vi "Spectrum_Main.vi"() -> ()   [LabVIEW 2021]
uses:
  Sources/Plotting-Axis.ctl
  GEN_States.ctl
  Sources/Config_Cluster.ctl
  Sources/Mode_Enum.ctl
  Sources/Data_Cluster.ctl
  Sources/Measurement_Cluster.ctl
  VISAS.ctl
  1375486a-d526-4950-a4e9-ede105372d37.vi
  <vilib>/Utility/config.llb/NI_LVConfig.lvlib
panel:
  in  "Control Tab":enum32{"General", "Scope/Gen", "VNA", "Configs"}(tab)
  out "VNA":bool
  out "Generator":bool
  in  "StopM_Button":bool
  in  "Log_Button":bool
  in  "Measure_Button":bool
  out "Globals":bool
  out "Scope":bool
  out "Logging":bool
  out "Measuring":bool
  out "Magnetic Field":dbl
  out "Temperature":dbl
  in  "Offset (V)":dbl
  in  "Amplitude (Vpp)":dbl
  in  "Frequency (Hz)":dbl
  in  "SendSet_scopgen_Button":bool
  in  "Refresh_scopgen_Button":bool
  in  "Vertical Scale (V/div)":dbl
  in  "Horizontal Scale (1/t)":dbl
  in  "Tab Control":enum32{"Scope", "Gen"}(tab)
  in  "Scope Channel":enum16{"Channel 1", "Channel 2"}(ring)
  in  "RTC1002 VISA COM":refnum<visa-resource-name>
  in  "Gen VISA COM":refnum<visa-resource-name>
  in  "LoadConfig_Button":bool
  in  "ApplyConfig_Button":bool
  in  "SaveConfig_Button":bool
  in  "Retry_Button":bool
  in  "Config Path (Blank is default)":path
  in  "Global Temp VAR":refnum<k21>
  in  "Global Mag VAR":refnum<k21>
  in  "Logging Path":path
  in  "Display Tab":T1(tab)
  out "Status":string
  in  "Clear_Button":bool
  in  "Y-Axis":T2
  in  "X-Axis":T2
  out "Test Graph":cluster{"X":dbl, "Y":dbl}[](graph)
  in  "Max Elements":i32=5000
  out "Scope Display":waveform(dbl)(graph)
  in  "Exit_Button":bool
  # "Instrument Settings"
  # "Global Var. Settings"
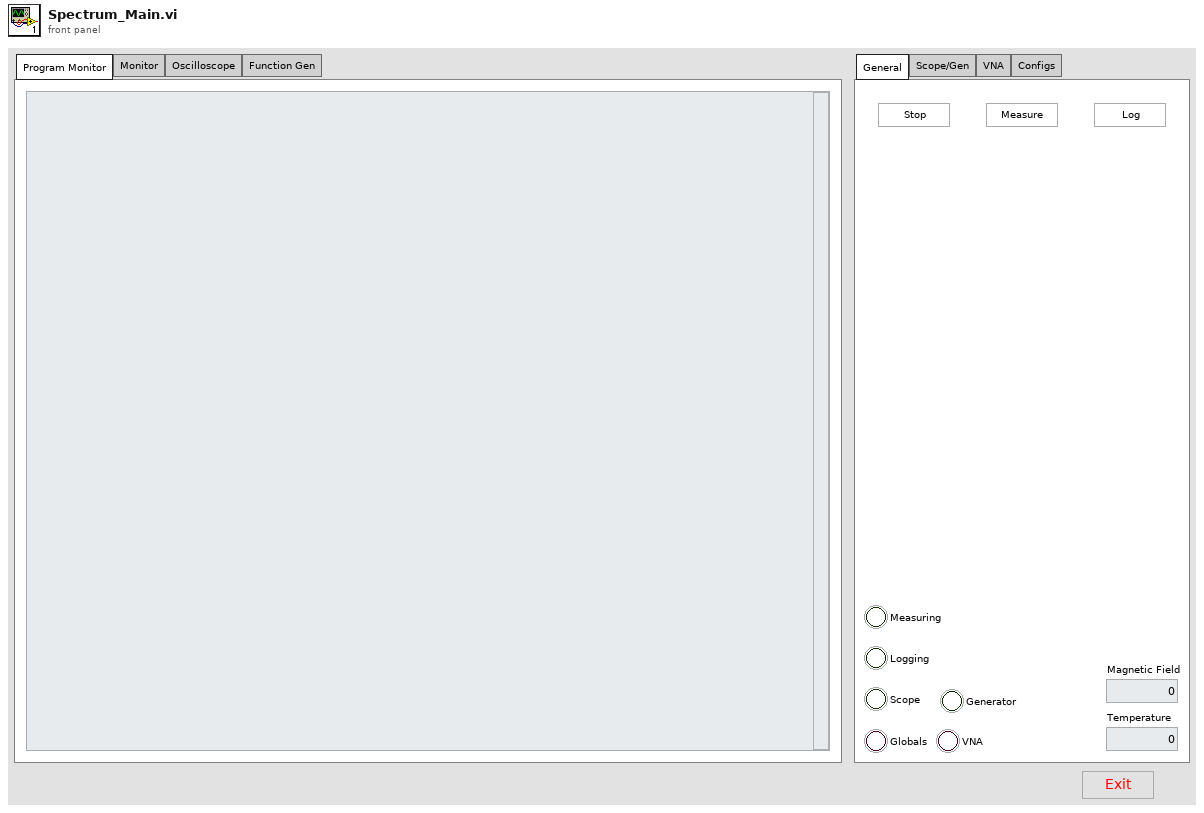
[diagram p1: front panel]
types:
  T1 = enum32{"Program Monitor", "Monitor", "Oscilloscope", "Function Gen"}
  T2 = typedef "Plotting-Axis.ctl" = enum16{"Time", "Temperature", "MagneticField", "Capacitance", "Loss"}
  T3 = typedef "GEN_States.ctl" = enum16{"SetupSettings", "GetSettings", "SetupInstruments", "SetupGEN", "SetupVNA", "ClearBuffers", "SwitchToMeas", "SwitchToLog", "SwitchToOff", "Disconnect", "ApplyConfig", "ExitSafe", "RefreshPlotMUnits", "UpdatePlots", "RefreshMUnits", "Read/WriteAll", "RetryComs", "SendSettings", "InitGUI", "RefreshGUI", "ComsFail", "SaveConfig", "Idle", "ProgInit"}
  T4 = typedef "VISAS.ctl" = cluster{"Gen VISA":refnum<visa-resource-name>, "RTC1002 VISA":refnum<visa-resource-name>, "VNA VISA":refnum<visa-resource-name>}
  T5 = typedef "Data_Cluster.ctl" = cluster{"Value":dbl, "GUI Data Cluster":cluster{"SBR":u16}, "Timing":cluster{"Last Operation":dbl}, "Measurements":T6[], "Scope Capture":waveform(dbl)}
  T6 = typedef "Measurement_Cluster.ctl" = cluster{"Time Stamp":timestamp, "Cap":dbl, "Temperature":dbl, "MagneticField":dbl, "Loss":dbl, "ExVoltage":dbl, "Error":dbl}
  T7 = typedef "Config_Cluster.ctl" = cluster{"General":cluster{"Config.ini":path, "Default Logging Path":path}, "Hardware":cluster{"Global T VAR":refnum<k21>, "Global B VAR":refnum<k21>, "VISAS":cluster{"GEN COM":refnum<visa-resource-name>, "SCOPE COM":refnum<visa-resource-name>, "VNA COM":refnum<visa-resource-name>}, "Connected?":cluster{"SCOPE":bool, "GEN":bool, "VNA":bool}}, "Operation":cluster{"Operation Mode":T8, "Status":string, "NewLog?":bool, "OvenWarn":bool, "Scope Settings":cluster{"TimeBase":dbl, "VerticalScale":dbl, "Channel":enum16{"Channel 2", "Channel 1"}}, "Gen Settings":cluster{"Amplitude":dbl, "Frequency":dbl, "Offset":dbl}}}
  T8 = typedef "Mode_Enum.ctl" = enum16{"Logging", "Idle-Off", "Idle"}
  T9 = cluster{"Scope":refnum<vi>, "Generator":refnum<vi>, "VNA":refnum<vi>}
  T10 = typedef "NI_LVConfig.lvlib/Config Data RefNum.ctl" = refnum<k1>
  T11 = cluster{"GEN COM":refnum<visa-resource-name>, "SCOPE COM":refnum<visa-resource-name>, "VNA COM":refnum<visa-resource-name>}
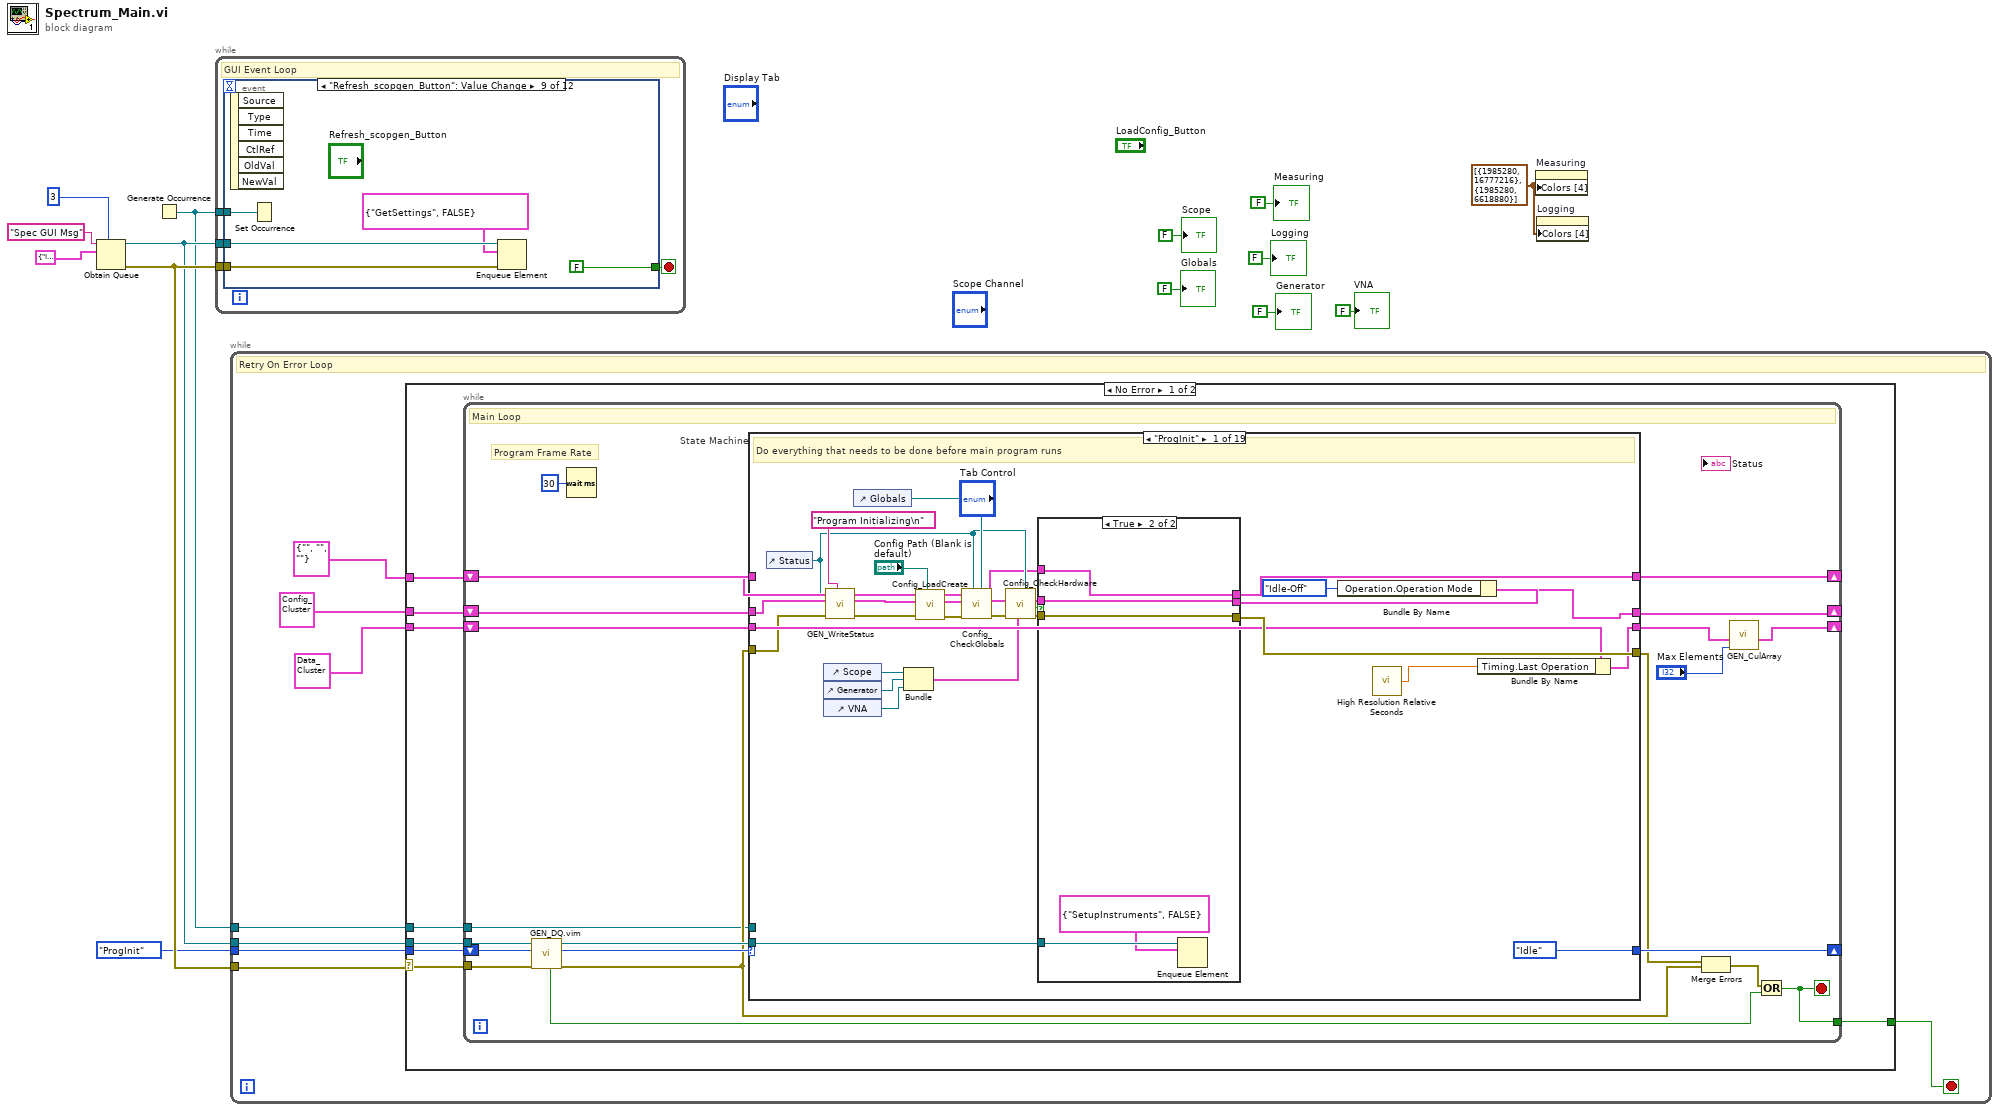
[diagram p0: block diagram]
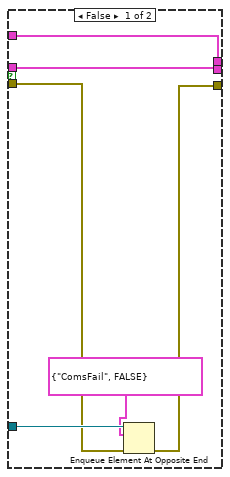
[diagram p2: hidden frame]
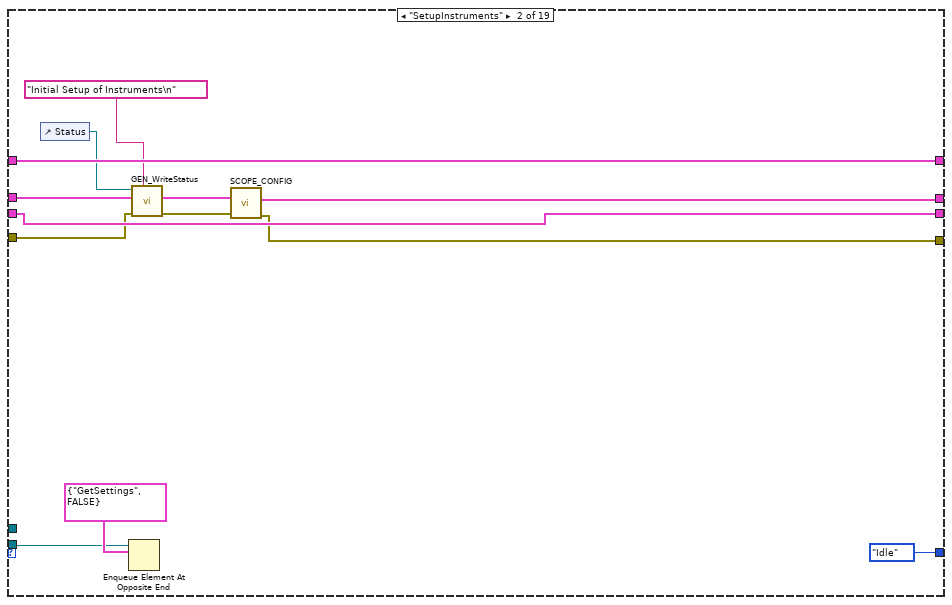
[diagram p3: hidden frame]
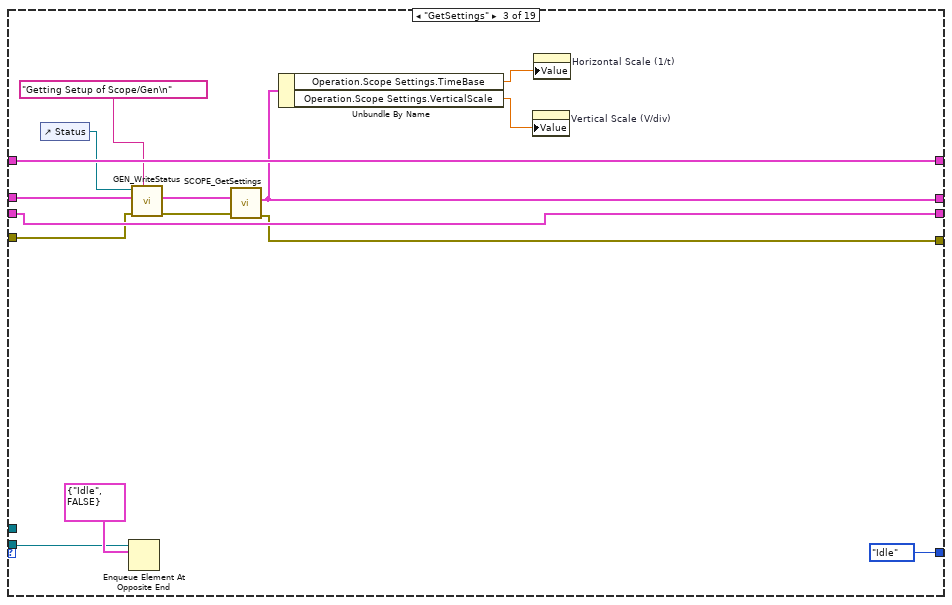
[diagram p4: hidden frame]
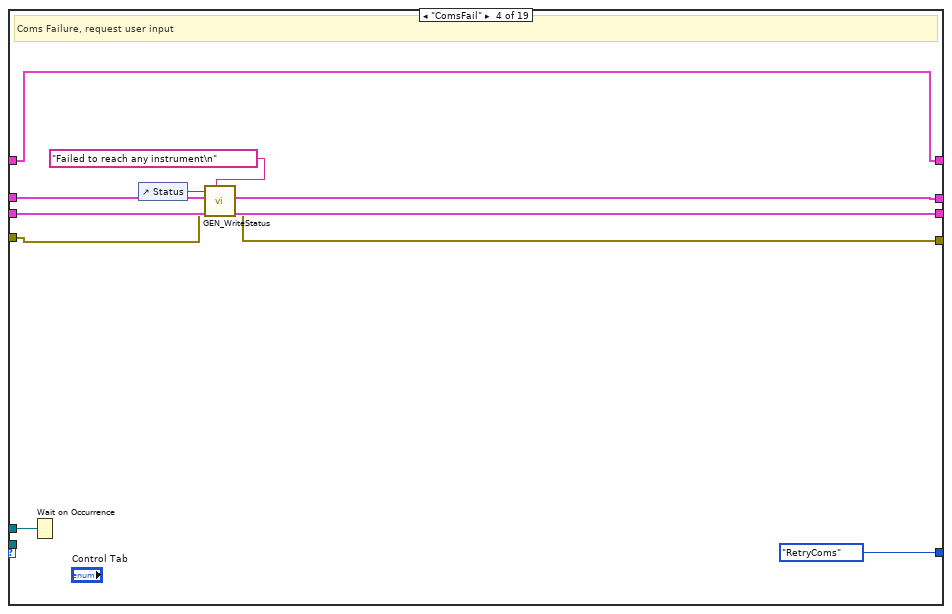
[diagram p5: hidden frame]
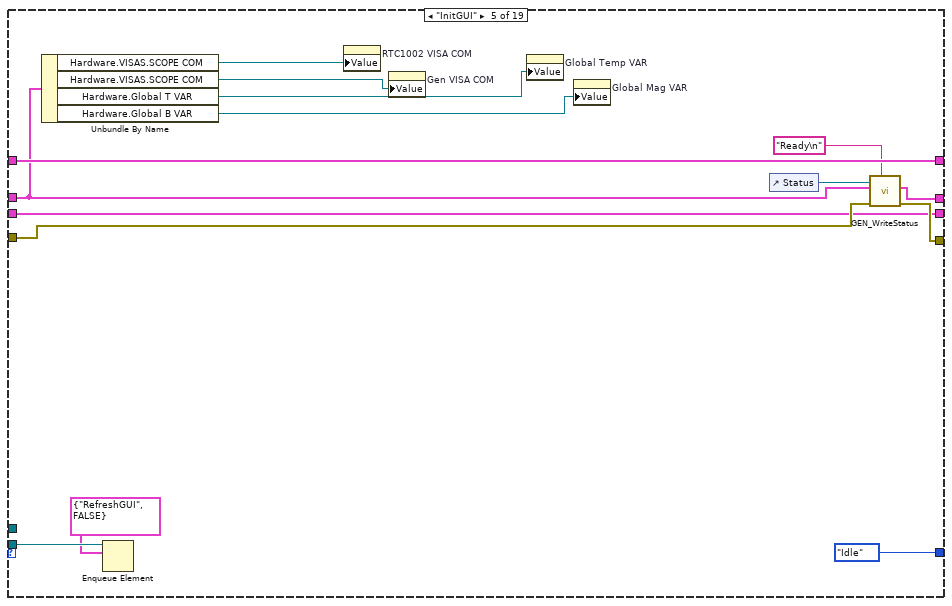
[diagram p6: hidden frame]
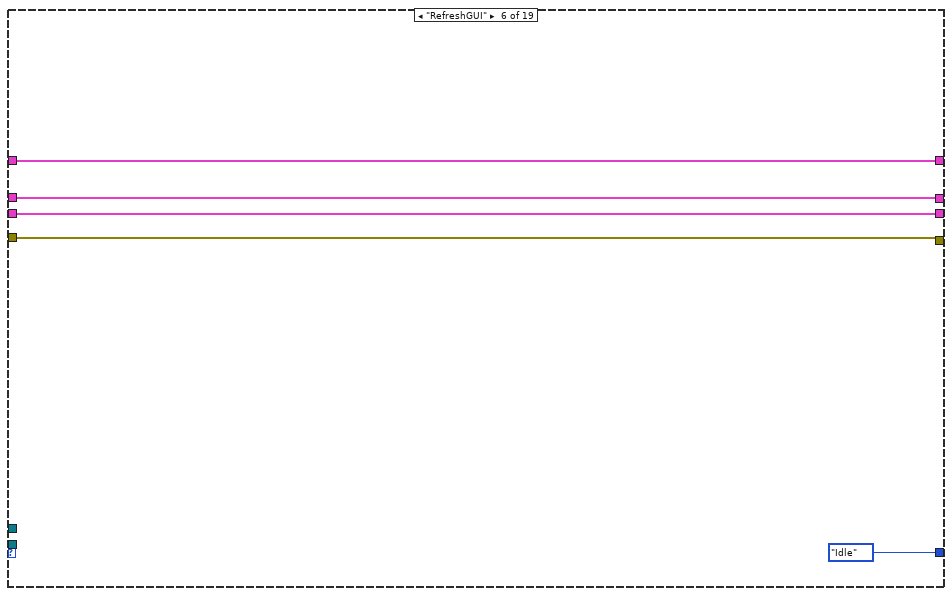
[diagram p7: hidden frame]
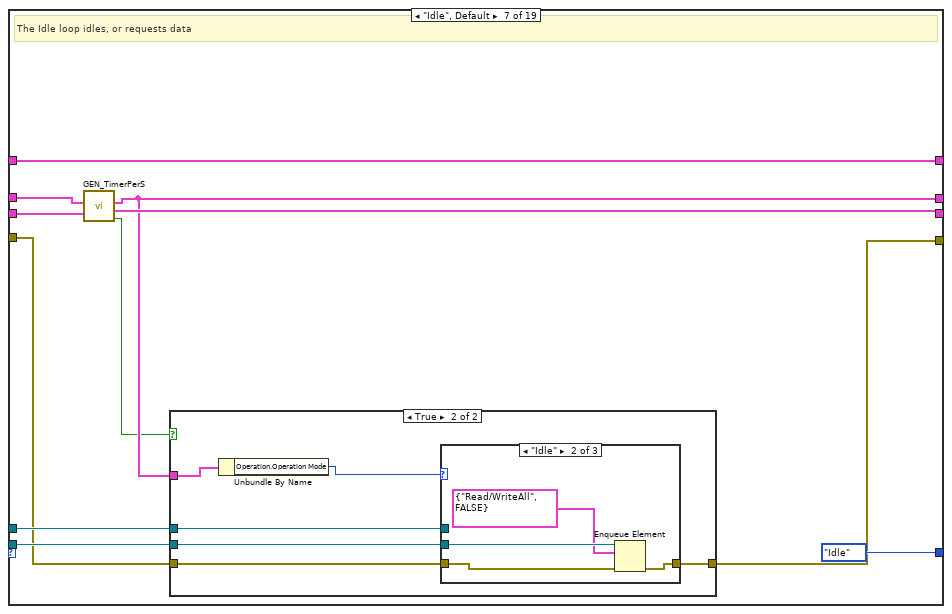
[diagram p8: hidden frame]
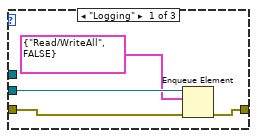
[diagram p10: hidden frame]
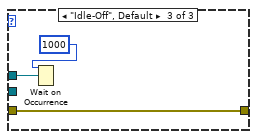
[diagram p11: hidden frame]
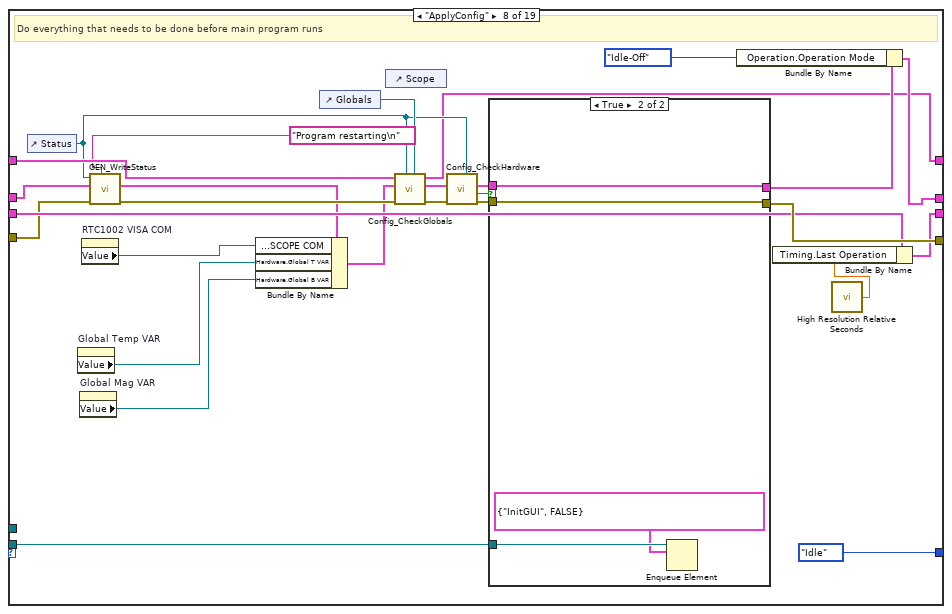
[diagram p12: hidden frame]
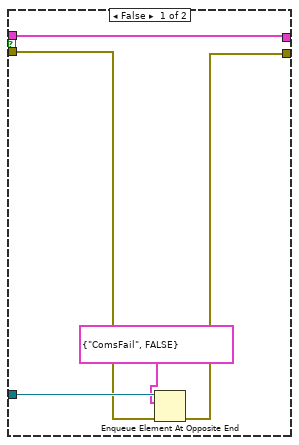
[diagram p13: hidden frame]
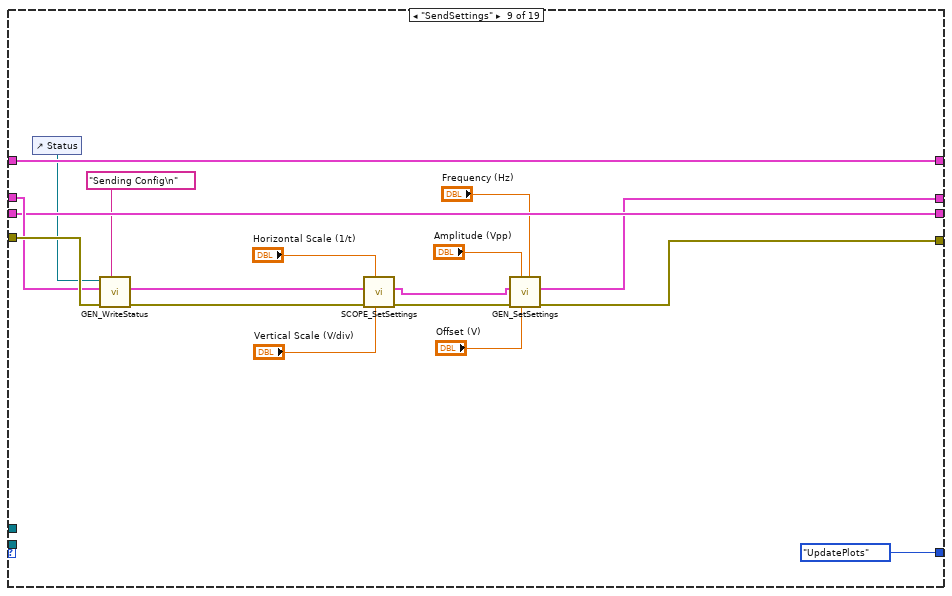
[diagram p14: hidden frame]
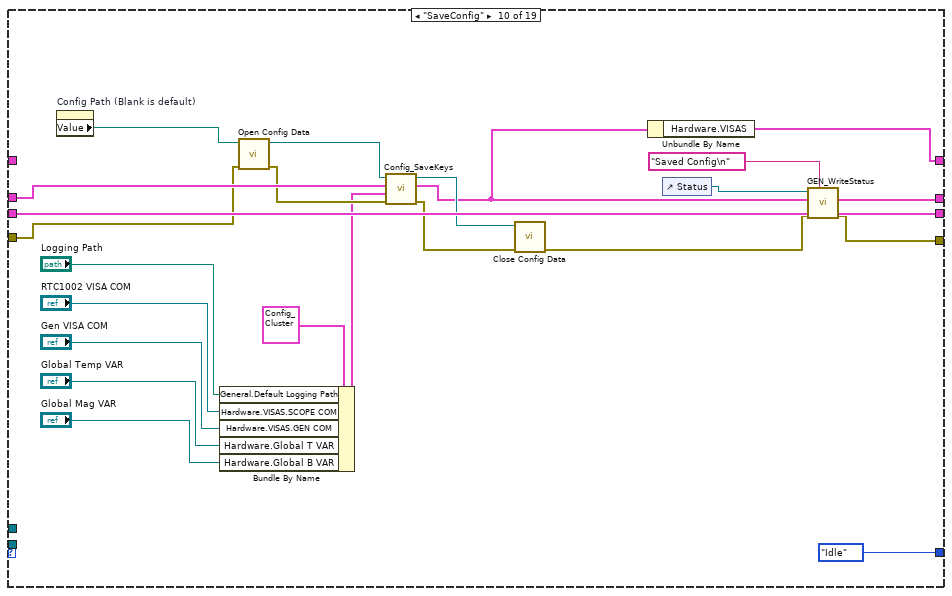
[diagram p15: hidden frame]
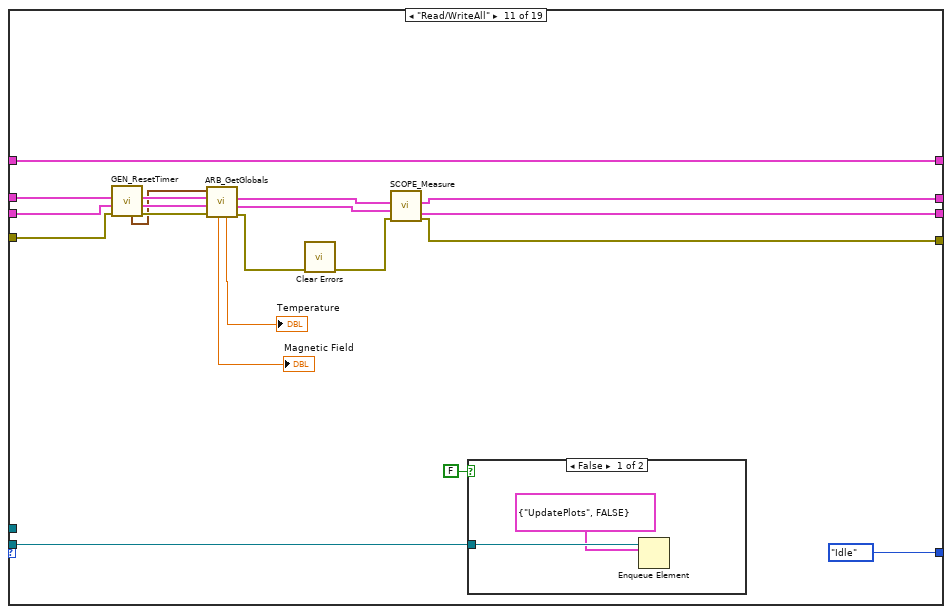
[diagram p16: hidden frame]
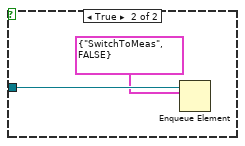
[diagram p17: hidden frame]
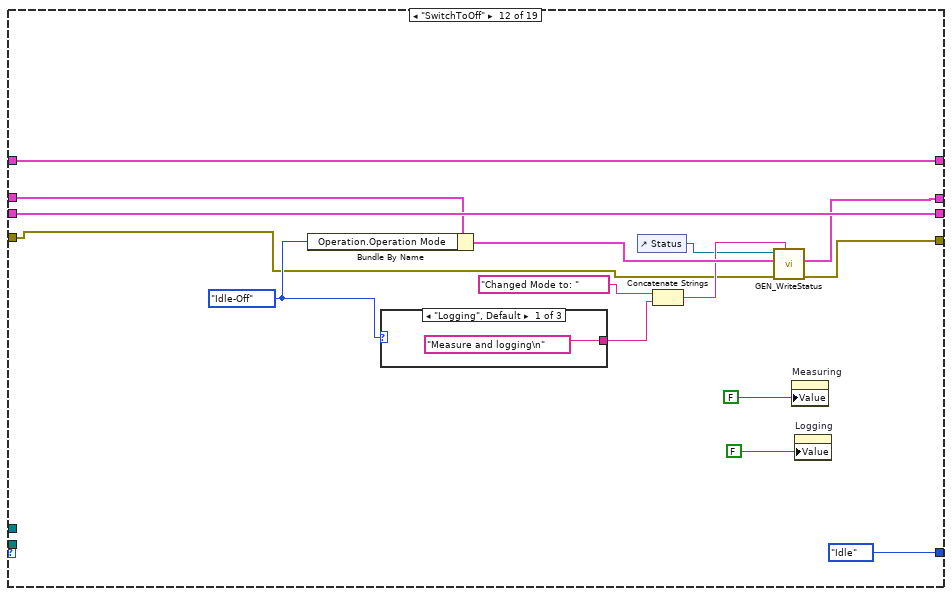
[diagram p18: hidden frame]
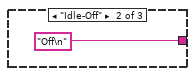
[diagram p19: hidden frame]
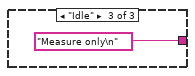
[diagram p20: hidden frame]
diagram:
  w3 = cluster{u32, u32}[] [{1985280, 16777216}, {1985280, 6618880}] ("Colors [4]")
  n1 = Obtain Queue(max queue size (-1, unlimited)=3, name (unnamed)="Spec GUI Msg", element data type=cluster{T3, bool} {enum."Idle", TRUE}) -> (queue out=w10:refnum<queue>, error out=w11:errorcluster)  [unwired: 2 in, 1 out]
  n2 = Generate Occurrence() -> (w8:refnum<k4>)
  n3 = while {
    tunnel: w10 -> [w18]
    tunnel: w11 -> [w17]
    tunnel: w8 -> [w15]
    stop <- w16 stop-if-true
    # "GUI Event Loop"
    n4 = event shown="[8] \"Refresh_scopgen_Button\": Value Change" {
      selector: _ -> [_ _ _ _ _ _ _ _ _ _ _ _]
      dyn-events: _ -> [_ _ _ _ _ _ _ _ _ _ _ _]
      timeout: _ -> [_ _ _ _ _ _ _ _ _ _ _ _]
      tunnel: w18 -> [_ w23 w28 w33 w38 w43 w48 w53 w58 w63 w68 w73]
      tunnel: w17 -> [_ w22 w27 w32 w37 w42 w47 w52 w57 w62 w67 w72]
      tunnel: [_ TRUE FALSE FALSE FALSE FALSE FALSE FALSE FALSE FALSE FALSE FALSE] -> w16
      tunnel: w15 -> [_ w19 w24 w29 w34 w39 w44 w49 w54 w59 w64 w69]
      event Timeout {
        n5 = event-data() -> ()  [unwired: 1 in, 3 out]
      }
      event "Exit_Button": Value Change {
        n6 = event-data() -> ()  [unwired: 1 in, 6 out]
        n7 = Set Occurrence(w19) -> ()
        n8 = Enqueue Element At Opposite End(queue=w23, element=cluster{T3, bool} {enum."ExitSafe", TRUE}, error in (no error)=w22) -> ()  [unwired: 1 in, 3 out]
      }
      event "Retry_Button": Value Change {
        n9 = event-data() -> ()  [unwired: 1 in, 6 out]
        n10 = Set Occurrence(w24) -> ()
        n11 = Enqueue Element At Opposite End(queue=w28, element=cluster{T3, bool} {enum."RetryComs", FALSE}, error in (no error)=w27) -> ()  [unwired: 1 in, 3 out]
      }
      event "ApplyConfig_Button": Value Change {
        n12 = event-data() -> ()  [unwired: 1 in, 6 out]
        n13 = Set Occurrence(w29) -> ()
        n14 = Enqueue Element(queue=w33, element=cluster{T3, bool} {enum."Disconnect", FALSE}, error in (no error)=w32) -> ()  [unwired: 1 in, 3 out]
      }
      event "SaveConfig_Button": Value Change {
        n15 = event-data() -> ()  [unwired: 1 in, 6 out]
        n16 = Set Occurrence(w34) -> ()
        n17 = Enqueue Element(queue=w38, element=cluster{T3, bool} {enum."SaveConfig", FALSE}, error in (no error)=w37) -> ()  [unwired: 1 in, 3 out]
      }
      event "StopM_Button": Value Change {
        n18 = event-data() -> ()  [unwired: 1 in, 6 out]
        n19 = Set Occurrence(w39) -> ()
        n20 = Enqueue Element(queue=w43, element=cluster{T3, bool} {enum."SwitchToOff", FALSE}, error in (no error)=w42) -> ()  [unwired: 1 in, 3 out]
      }
      event "Measure_Button": Value Change {
        n21 = event-data() -> ()  [unwired: 1 in, 6 out]
        n22 = Set Occurrence(w44) -> ()
        n23 = Enqueue Element(queue=w48, element=cluster{T3, bool} {enum."SwitchToMeas", FALSE}, error in (no error)=w47) -> ()  [unwired: 1 in, 3 out]
      }
      event "SendSet_scopgen_Button": Value Change {
        n24 = event-data() -> ()  [unwired: 1 in, 6 out]
        n25 = Set Occurrence(w49) -> ()
        n26 = Enqueue Element(queue=w53, element=cluster{T3, bool} {enum."SendSettings", FALSE}, error in (no error)=w52) -> ()  [unwired: 1 in, 3 out]
      }
      event "Refresh_scopgen_Button": Value Change {
        n27 = event-data() -> ()  [unwired: 1 in, 6 out]
        n28 = Set Occurrence(w54) -> ()
        n29 = Enqueue Element(queue=w58, element=cluster{T3, bool} {enum."GetSettings", FALSE}, error in (no error)=w57) -> ()  [unwired: 1 in, 3 out]
      }
      event "Log_Button": Value Change {
        n30 = event-data() -> ()  [unwired: 1 in, 6 out]
        n31 = Set Occurrence(w59) -> ()
        n32 = Enqueue Element(queue=w63, element=cluster{T3, bool} {enum."SwitchToLog", FALSE}, error in (no error)=w62) -> ()  [unwired: 1 in, 3 out]
      }
      event "Clear_Button": Value Change {
        n33 = event-data() -> ()  [unwired: 1 in, 6 out]
        n34 = Set Occurrence(w64) -> ()
        n35 = Enqueue Element(queue=w68, element=cluster{T3, bool} {enum."ClearBuffers", FALSE}, error in (no error)=w67) -> ()  [unwired: 1 in, 3 out]
      }
      event Value Change {
        n36 = event-data() -> ()  [unwired: 1 in, 6 out]
        n37 = Set Occurrence(w69) -> ()
        n38 = Enqueue Element(queue=w73, element=cluster{T3, bool} {enum."RefreshPlotMUnits", FALSE}, error in (no error)=w72) -> ()  [unwired: 1 in, 3 out]
      }
    }
  }
  n39 = while {
    tunnel: w11 -> [w81]
    tunnel: w10 -> [w80]
    tunnel: GEN_States."ProgInit" ("State") -> [w79]
    tunnel: w8 -> [w75]
    stop <- w78 stop-if-true
    # "Retry On Error Loop"
    n40 = case shown="No Error" w81 {
      selector: w81 -> [w89 _]
      tunnel: w80 -> [w88 _]
      tunnel: w79 -> [w82 _]
      tunnel: [w87 TRUE] -> w78
      tunnel: T4 {"Gen VISA"="", "RTC1002 VISA"="", "VNA VISA"=""} -> [w86 _]
      tunnel: T7 {"General"={"Config.ini"=path "", "Default Logging Path"=path ""}, "Hardware"={"Global T VAR"="", "Global B VAR"="", "VISAS"={"GEN COM"="", "SCOPE COM"="", "VNA COM"=""}, "Connected?"={"SCOPE"=FALSE, "GEN"=FALSE, "VNA"=FALSE}}, "Operation"={"Operation Mode"=enum."Logging", "Status"="", "NewLog?"=FALSE, "OvenWarn"=FALSE, "Scope Settings"={"TimeBase"=0.0, "VerticalScale"=0.0, "Channel"=enum."Channel 2"}, "Gen Settings"={"Amplitude"=0.0, "Frequency"=0.0, "Offset"=0.0}}} -> [w85 _]
      tunnel: T5 {"Value"=0.0, "GUI Data Cluster"={"SBR"=0}, "Timing"={"Last Operation"=0.0}, "Measurements"=[], "Scope Capture"={"t0"=timestamp(0 s since 1904-01-01), "dt"=1.0, "Y"=[]}} -> [w84 _]
      tunnel: w75 -> [w83 _]
      frame No Error {
        n41 = while {
          tunnel: w89 -> [w109]
          tunnel: w88 -> [w108]
          shift-right: [w101] -> _
          shift-left: w82 -> [w107]
          tunnel: [w103] -> w87
          shift-right: [w100] -> _
          shift-left: w86 -> [w102]
          shift-right: [w97] -> _
          shift-left: w85 -> [w98]
          shift-right: [w91] -> _
          shift-left: w84 -> [w96]
          tunnel: w83 -> [w93]
          stop <- w103 stop-if-true
          # "Program Frame Rate"
          # "Main Loop"
          n42 = call "GEN_DQ.vim"("error in (no error)"=w109, "Variant"=w107, "queue In"=w108) -> ("error out"=w95:errorcluster, "Variant Out"=w106:T3, "queue out"=w99:refnum<queue>, "Exit?"=w104:bool)  [unwired: 5 in]
          n43 = Wait (ms)(milliseconds to wait=u32 30) -> ()  [unwired: 1 out]
          n44 = case "State Machine" shown="\"ProgInit\"" w106 {
            tunnel: w102 -> [w140 w166 w181 w185 w206 w210 w222 w266 w294 _ w337 w356 w374 w400 w420 w428 w434 w459 w478]
            tunnel: [GEN_States."Idle" ("State") GEN_States."Idle" ("State") GEN_States."Idle" ("State") GEN_States."RetryComs" ("State") GEN_States."Idle" ("State") GEN_States."Idle" ("State") GEN_States."Idle" ("State") GEN_States."Idle" ("State") GEN_States."UpdatePlots" ("State") GEN_States."Idle" ("State") GEN_States."Idle" ("State") GEN_States."Idle" ("State") GEN_States."Idle" ("State") w386 GEN_States."Idle" ("State") GEN_States."Idle" ("State") GEN_States."Idle" ("State") GEN_States."Idle" ("State") GEN_States."ExitSafe" ("State")] -> w101
            tunnel: [w135 w166 w181 w185 w206 w210 w222 w242 w294 w295 w337 w356 w374 w400 w420 w428 w434 w459 w478] -> w100
            tunnel: w99 -> [w134 w162 w177 _ w204 _ w219 w261 _ _ w330 _ _ _ _ _ _ w443 _]
            tunnel: w98 -> [w126 w161 w176 w187 w201 w207 w216 w253 w291 w315 w329 w354 w372 w398 w419 w425 w433 w454 w472]
            tunnel: [w127 w155 w169 w186 w200 w207 w213 w254 w281 w308 w322 w351 w369 w387 w419 w425 w433 w453 w471] -> w97
            tunnel: w96 -> [w133 w165 w180 w190 w193 w208 w215 w260 w290 w317 w328 w355 w373 w399 w410 w426 w431 w458 w477]
            tunnel: [w132 w165 w180 w190 w193 w208 w214 w259 w290 w317 w321 w355 w373 w399 w412 w426 w430 w458 w477] -> w92
            tunnel: w95 -> [w124 w160 w175 w182 w198 w209 w218 w252 w292 w314 w326 w346 w364 w392 w415 w424 w432 w452 w470]
            tunnel: [w136 w154 w170 w188 w197 w209 w217 w262 w280 w304 w320 w345 w363 w391 w415 w424 w432 w451 w469] -> w94
            tunnel: w93 -> [_ _ _ w189 _ _ w220 _ _ _ _ _ _ _ _ _ _ _ _]
            frame "ProgInit" {
              # "Do everything that needs to be done before main program runs"
              n45 = control-ref of="Status"() -> (w116:refnum<vi>)
              n46 = control-ref of="Scope"() -> (w114:refnum<vi>)
              n47 = control-ref of="Generator"() -> (w113:refnum<vi>)
              n48 = control-ref of="VNA"() -> (w112:refnum<vi>)
              n49 = call "GEN_WriteStatus.vi"("Input String"="Program Initializing\n" ("Status"), "error in (no error)"=w124, "Config_Cluster"=w126, "Status Ref"=w116) -> ("error out"=w123:errorcluster, "Config_Cluster Out"=w125:T7)  [unwired: 6 in]
              n50 = control-ref of="Globals"() -> (w117:refnum<vi>)
              n51 = Bundle("Scope"=w114, "Generator"=w113, "VNA"=w112) -> (w111:T9)  [unwired: 1 in]
              n52 = call "Config_LoadCreate.vi"("Config In"="Config Path (Blank is default)", "error In"=w123, "Configuration Cluster"=w125, 11:w140) -> ("error out"=w119:errorcluster, "Configuration Cluster Out"=w120:T7, 3:w122:T4)  [unwired: 5 in]
              n53 = call "Config_CheckGlobals.vi"("GlobalsLED Ref"=w117, "Status Ref"=w116, "error in (no error)"=w119, "Config Cluster"=w120, "VISAS"=w122) -> ("error out"=w118:errorcluster, "Config Cluster Out"=w121:T7, "VISAS"=w115:T4)  [unwired: 4 in]
              n54 = call "Config_CheckHardware.vi"("Status Ref"=w116, "Ref Cluster"=w111, "error in (no error)"=w118, "Config Cluster"=w121) -> ("error out"=w138:errorcluster, "Connected?"=w139:bool, "Config Cluster Out"=w137:T7)  [unwired: 5 in]
              n55 = case shown="True" w139 {
                tunnel: w138 -> [w144 w152]
                tunnel: w137 -> [w147 w153]
                tunnel: w115 -> [w148 w149]
                tunnel: [w148 w149] -> w135
                tunnel: [w147 w153] -> w130
                tunnel: [w143 w152] -> w136
                tunnel: w134 -> [w146 w151]
                frame False {
                  n56 = Enqueue Element At Opposite End(queue=w146, element=cluster{T3, bool} {enum."ComsFail", FALSE}, error in (no error)=w144) -> (error out=w143:errorcluster)  [unwired: 1 in, 2 out]
                }
                frame True {
                  n57 = Enqueue Element(queue=w151, element=cluster{T3, bool} {enum."SetupInstruments", FALSE}) -> ()  [unwired: 2 in, 3 out]
                }
              }
              n58 = Bundle By Name(cluster=w130, "Operation.Operation Mode"=Mode_Enum."Idle-Off") -> (w127:T7)
              n59 = call <vilib>:"High Resolution Relative Seconds.vi"() -> ("relative seconds"=w131:dbl)
              n60 = Bundle By Name(cluster=w133, "Timing.Last Operation"=w131) -> (w132:T5)
            }
            frame "SetupInstruments" {
              n61 = control-ref of="Status"() -> (w159:refnum<vi>)
              n62 = Enqueue Element At Opposite End(queue=w162, element=cluster{T3, bool} {enum."GetSettings", FALSE}) -> ()  [unwired: 2 in, 3 out]
              n63 = call "GEN_WriteStatus.vi"("Input String"="Initial Setup of Instruments\n", "error in (no error)"=w160, "Config_Cluster"=w161, "Status Ref"=w159) -> ("error out"=w156:errorcluster, "Config_Cluster Out"=w157:T7)  [unwired: 6 in]
              n64 = call "SCOPE_CONFIG.vi"("error in (no error)"=w156, "Configuration Cluster"=w157) -> ("error out"=w154:errorcluster, "Configuration Cluster Out"=w155:T7)  [unwired: 8 in]
            }
            frame "GetSettings" {
              n65 = control-ref of="Status"() -> (w174:refnum<vi>)
              n66 = Enqueue Element At Opposite End(queue=w177, element=cluster{T3, bool} {enum."Idle", FALSE}) -> ()  [unwired: 2 in, 3 out]
              n67 = call "GEN_WriteStatus.vi"("Input String"="Getting Setup of Scope/Gen\n", "error in (no error)"=w175, "Config_Cluster"=w176, "Status Ref"=w174) -> ("error out"=w171:errorcluster, "Config_Cluster Out"=w172:T7)  [unwired: 6 in]
              n68 = call "SCOPE_GetSettings.vi"("error in (no error)"=w171, "Configuration Cluster"=w172) -> ("error out"=w170:errorcluster, "Configuration Cluster Out"=w169:T7)  [unwired: 8 in]
              n69 = Unbundle By Name(w169) -> ("Operation.Scope Settings.TimeBase"=w168:dbl, "Operation.Scope Settings.VerticalScale"=w167:dbl)
              n70 = property on="Vertical Scale (V/div)" class="DigNum (strict)"("Value"=w167) -> ()  [unwired: 2 in, 2 out]
              n71 = property on="Horizontal Scale (1/t)" class="DigNum (strict)"("Value"=w168) -> ()  [unwired: 2 in, 2 out]
            }
            frame "ComsFail" {
              # "Coms Failure, request user input"
              n72 = Wait on Occurrence(2:w189) -> ()  [unwired: 2 in, 1 out]
              n73 = control-ref of="Status"() -> (w183:refnum<vi>)
              n74 = call "GEN_WriteStatus.vi"("Input String"="Failed to reach any instrument\n", "error in (no error)"=w182, "Config_Cluster"=w187, "Status Ref"=w183) -> ("error out"=w188:errorcluster, "Config_Cluster Out"=w186:T7)  [unwired: 6 in]
            }
            frame "InitGUI" {
              n75 = Unbundle By Name(w201) -> ("Hardware.VISAS.SCOPE COM"=w202:refnum<visa-resource-name>, "Hardware.VISAS.SCOPE COM"=w192:refnum<visa-resource-name>, "Hardware.Global T VAR"=w195:refnum<k21>, "Hardware.Global B VAR"=w194:refnum<k21>)
              n76 = Enqueue Element(queue=w204, element=cluster{T3, bool} {enum."RefreshGUI", FALSE}) -> ()  [unwired: 2 in, 3 out]
              n77 = property on="RTC1002 VISA COM" class="VISAName"("Value"=w202) -> ()  [unwired: 2 in, 2 out]
              n78 = property on="Gen VISA COM" class="VISAName"("Value"=w192) -> ()  [unwired: 2 in, 2 out]
              n79 = property on="Global Temp VAR" class="Variable (strict)"("Value"=w195) -> ()  [unwired: 2 in, 2 out]
              n80 = property on="Global Mag VAR" class="Variable (strict)"("Value"=w194) -> ()  [unwired: 2 in, 2 out]
              n81 = control-ref of="Status"() -> (w196:refnum<vi>)
              n82 = call "GEN_WriteStatus.vi"("Input String"="Ready\n", "error in (no error)"=w198, "Config_Cluster"=w201, "Status Ref"=w196) -> ("error out"=w197:errorcluster, "Config_Cluster Out"=w200:T7)  [unwired: 6 in]
            }
            frame "RefreshGUI" {
            }
            frame "Idle", Default {
              # "The Idle loop idles, or requests data"
              n83 = call "GEN_TimerPerS.vi"("Data_In"=w215, "Config_In"=w216) -> ("Time"=w212:bool, "Data_In 2"=w214:T5, "Config_In 2"=w213:T7)  [unwired: 7 in]
              n84 = case shown="True" w212 {
                tunnel: w220 -> [_ w229]
                tunnel: w219 -> [_ w228]
                tunnel: w218 -> [w223 w227]
                tunnel: [w223 w226] -> w217
                tunnel: w213 -> [_ w225]
                frame False {
                }
                frame True {
                  n85 = Unbundle By Name(w225) -> ("Operation.Operation Mode"=w224:T8)
                  n86 = case shown="\"Idle\"" w224 {
                    tunnel: w229 -> [_ _ w240]
                    tunnel: w228 -> [w233 w237 _]
                    tunnel: w227 -> [w232 w236 w239]
                    tunnel: [w230 w234 w239] -> w226
                    frame "Logging" {
                      n87 = Enqueue Element(queue=w233, element=cluster{T3, bool} {enum."Read/WriteAll", FALSE}, error in (no error)=w232) -> (error out=w230:errorcluster)  [unwired: 1 in, 2 out]
                    }
                    frame "Idle" {
                      n88 = Enqueue Element(queue=w237, element=cluster{T3, bool} {enum."Read/WriteAll", FALSE}, error in (no error)=w236) -> (error out=w234:errorcluster)  [unwired: 1 in, 2 out]
                    }
                    frame "Idle-Off", Default {
                      n89 = Wait on Occurrence(2:w240, 3:1000 ("ms timeout (-1)")) -> ()  [unwired: 1 in, 1 out]
                    }
                  }
                }
              }
            }
            frame "ApplyConfig" {
              # "Do everything that needs to be done before main program runs"
              n90 = control-ref of="Status"() -> (w243:refnum<vi>)
              n91 = property on="Global Temp VAR" class="Variable (strict)"() -> ("Value"=w246:refnum<k21>)  [unwired: 2 in, 2 out]
              n92 = property on="Global Mag VAR" class="Variable (strict)"() -> ("Value"=w245:refnum<k21>)  [unwired: 2 in, 2 out]
              n93 = property on="RTC1002 VISA COM" class="VISAName"() -> ("Value"=w241:refnum<visa-resource-name>)  [unwired: 2 in, 2 out]
              n94 = call "GEN_WriteStatus.vi"("Input String"="Program restarting\n" ("Status"), "error in (no error)"=w252, "Config_Cluster"=w253, "Status Ref"=w243) -> ("error out"=w251:errorcluster, "Config_Cluster Out"=w248:T7)  [unwired: 6 in]
              n95 = Bundle By Name(cluster=w248, "Hardware.VISAS.SCOPE COM"=w241, "Hardware.Global T VAR"=w246, "Hardware.Global B VAR"=w245) -> (w247:T7)
              n96 = control-ref of="Globals"() -> (w244:refnum<vi>)
              n97 = control-ref of="Scope"() -> ()  [unwired: 1 out]
              n98 = call "Config_CheckGlobals.vi"("GlobalsLED Ref"=w244, "Status Ref"=w243, "error in (no error)"=w251, "Config Cluster"=w247, "VISAS"=w266) -> ("error out"=w249:errorcluster, "Config Cluster Out"=w250:T7, "VISAS"=w242:T4)  [unwired: 4 in]
              n99 = call "Config_CheckHardware.vi"("Status Ref"=w243, "error in (no error)"=w249, "Config Cluster"=w250) -> ("error out"=w264:errorcluster, "Connected?"=w265:bool, "Config Cluster Out"=w263:T7)  [unwired: 6 in]
              n100 = case shown="True" w265 {
                tunnel: w264 -> [w269 w275]
                tunnel: w263 -> [w272 w276]
                tunnel: [w272 w276] -> w257
                tunnel: [w268 w275] -> w262
                tunnel: w261 -> [w271 w274]
                frame False {
                  n101 = Enqueue Element At Opposite End(queue=w271, element=cluster{T3, bool} {enum."ComsFail", FALSE}, error in (no error)=w269) -> (error out=w268:errorcluster)  [unwired: 1 in, 2 out]
                }
                frame True {
                  n102 = Enqueue Element(queue=w274, element=cluster{T3, bool} {enum."InitGUI", FALSE}) -> ()  [unwired: 2 in, 3 out]
                }
              }
              n103 = Bundle By Name(cluster=w257, "Operation.Operation Mode"=Mode_Enum."Idle-Off") -> (w254:T7)
              n104 = call <vilib>:"High Resolution Relative Seconds.vi"() -> ("relative seconds"=w258:dbl)
              n105 = Bundle By Name(cluster=w260, "Timing.Last Operation"=w258) -> (w259:T5)
            }
            frame "SendSettings" {
              n106 = control-ref of="Status"() -> (w289:refnum<vi>)
              n107 = call "GEN_WriteStatus.vi"("Input String"="Sending Config\n", "error in (no error)"=w292, "Config_Cluster"=w291, "Status Ref"=w289) -> ("error out"=w286:errorcluster, "Config_Cluster Out"=w287:T7)  [unwired: 6 in]
              n108 = call "SCOPE_SetSettings.vi"("Vertical Scale (0.005)"="Vertical Scale (V/div)", "Time Scale (100.0e-6)"="Horizontal Scale (1/t)", "error in (no error)"=w286, "Configuration Cluster"=w287) -> ("error out"=w282:errorcluster, "Configuration Cluster Out"=w283:T7)  [unwired: 6 in]
              n109 = call "GEN_SetSettings.vi"("Frequency (1000 Hz)"="Frequency (Hz)", "DC Offset (0.00 V)"="Offset (V)", "Amplitude (1.0 Vpp)"="Amplitude (Vpp)", "error in (no error)"=w282, "Configuration Cluster"=w283) -> ("error out"=w280:errorcluster, "Configuration Cluster Out"=w281:T7)  [unwired: 5 in]
            }
            frame "SaveConfig" {
              n110 = property on="Config Path (Blank is default)" class="Path"() -> ("Value"=w309:path)  [unwired: 2 in, 2 out]
              n111 = Bundle By Name(cluster=T7 {"General"={"Config.ini"=path "", "Default Logging Path"=path ""}, "Hardware"={"Global T VAR"="", "Global B VAR"="", "VISAS"={"GEN COM"="", "SCOPE COM"="", "VNA COM"=""}, "Connected?"={"SCOPE"=FALSE, "GEN"=FALSE, "VNA"=FALSE}}, "Operation"={"Operation Mode"=enum."Idle-Off", "Status"="", "NewLog?"=FALSE, "OvenWarn"=FALSE, "Scope Settings"={"TimeBase"=0.0, "VerticalScale"=0.0, "Channel"=enum."Channel 2"}, "Gen Settings"={"Amplitude"=0.0, "Frequency"=0.0, "Offset"=0.0}}} ("Configuration Save"), "General.Default Logging Path"="Logging Path", "Hardware.VISAS.SCOPE COM"="RTC1002 VISA COM", "Hardware.VISAS.GEN COM"="Gen VISA COM", "Hardware.Global T VAR"="Global Temp VAR", "Hardware.Global B VAR"="Global Mag VAR") -> (w302:T7)
              n112 = call <vilib>:"Open Config Data.vi"("error in (no error)"=w314, "configuration file path"=w309) -> ("error out"=w313:errorcluster, "refnum"=w312:T10)  [unwired: 7 in, 1 out]
              n113 = call "Config_SaveKeys.vi"("error in (no error)"=w313, "Configuration Save"=w302, "Configuration Cluster"=w315, "Config In"=w312) -> ("error out"=w310:errorcluster, "output cluster"=w296:T7, "refnum out"=w311:T10)  [unwired: 5 in]
              n114 = call <vilib>:"Close Config Data.vi"("error in (no error)"=w310, "refnum"=w311) -> ("error out"=w305:errorcluster)  [unwired: 8 in, 1 out]
              n115 = Unbundle By Name(w296) -> ("Hardware.VISAS"=w295:T11)
              n116 = control-ref of="Status"() -> (w306:refnum<vi>)
              n117 = call "GEN_WriteStatus.vi"("Input String"="Saved Config\n", "error in (no error)"=w305, "Config_Cluster"=w296, "Status Ref"=w306) -> ("error out"=w304:errorcluster, "Config_Cluster Out"=w308:T7)  [unwired: 6 in]
            }
            frame "Read/WriteAll" {
              n118 = call "GEN_ResetTimer.vi"("error in (no error)"=w326, "Data_In"=w328, "Cluster IN"=w329) -> ("error out"=w333:errorcluster, "Data_In 2"=w334:T5, "Cluster OUT"=w335:T7, "TimeStamp"=w327:timestamp)  [unwired: 5 in]
              n119 = call "ARB_GetGlobals.vi"("error in (no error)"=w333, "Data_In"=w334, "Cluster IN"=w335, "Start Stamp"=w327) -> ("error out"=w318:errorcluster, "Data_Out"=w324:T5, "Cluster OUT"=w323:T7, "T Var"=→"Temperature":dbl, "B Var"=→"Magnetic Field":dbl)  [unwired: 1 in, 2 out]
              n120 = call <vilib>:"Clear Errors.vi"("error in (no error)"=w318) -> ("error out"=w319:errorcluster)  [unwired: 5 in, 1 out]
              n121 = call "SCOPE_Measure.vi"("error in (no error)"=w319, "Data Cluster"=w324, "Configuration Cluster"=w323) -> ("error out"=w320:errorcluster, "Data Cluster out"=w321:T5, "Configuration Cluster Out"=w322:T7)  [unwired: 6 in]
              n122 = case shown="False" FALSE {
                tunnel: w330 -> [w339 w341]
                frame False {
                  n123 = Enqueue Element(queue=w339, element=cluster{T3, bool} {enum."UpdatePlots", FALSE}) -> ()  [unwired: 2 in, 3 out]
                }
                frame True {
                  n124 = Enqueue Element(queue=w341, element=cluster{T3, bool} {enum."SwitchToMeas", FALSE}) -> ()  [unwired: 2 in, 3 out]
                }
              }
            }
            frame "SwitchToOff" {
              w350 = Mode_Enum."Idle-Off" ("Operation.Operation Mode")
              n125 = Bundle By Name(cluster=w354, "Operation.Operation Mode"=w350) -> (w352:T7)
              n126 = case shown="\"Logging\", Default" w350 {
                tunnel: ["Measure and logging\n" "Off\n" "Measure only\n"] -> w349
                frame "Logging", Default {
                }
                frame "Idle-Off" {
                }
                frame "Idle" {
                }
              }
              n127 = control-ref of="Status"() -> (w344:refnum<vi>)
              n128 = Concatenate Strings("Changed Mode to: " ("string"), w349) -> (w347:string)
              n129 = call "GEN_WriteStatus.vi"("Input String"=w347, "error in (no error)"=w346, "Config_Cluster"=w352, "Status Ref"=w344) -> ("error out"=w345:errorcluster, "Config_Cluster Out"=w351:T7)  [unwired: 6 in]
              n130 = property on="Measuring" class="Bool (strict)"("Value"=FALSE ("Measuring")) -> ()  [unwired: 2 in, 2 out]
              n131 = property on="Logging" class="Bool (strict)"("Value"=FALSE ("Logging")) -> ()  [unwired: 2 in, 2 out]
            }
            frame "SwitchToMeas" {
              w368 = Mode_Enum."Idle" ("Operation.Operation Mode")
              n132 = Bundle By Name(cluster=w372, "Operation.Operation Mode"=w368) -> (w370:T7)
              n133 = case shown="\"Idle\"" w368 {
                tunnel: ["Measure and logging\n" "Off\n" "Measure only\n"] -> w367
                frame "Logging", Default {
                }
                frame "Idle-Off" {
                }
                frame "Idle" {
                }
              }
              n134 = control-ref of="Status"() -> (w362:refnum<vi>)
              n135 = Concatenate Strings("Changed Mode to: " ("string"), w367) -> (w365:string)
              n136 = call "GEN_WriteStatus.vi"("Input String"=w365, "error in (no error)"=w364, "Config_Cluster"=w370, "Status Ref"=w362) -> ("error out"=w363:errorcluster, "Config_Cluster Out"=w369:T7)  [unwired: 6 in]
              n137 = property on="Measuring" class="Bool (strict)"("Value"=TRUE ("Measuring")) -> ()  [unwired: 2 in, 2 out]
              n138 = property on="Logging" class="Bool (strict)"("Value"=FALSE ("Logging")) -> ()  [unwired: 2 in, 2 out]
            }
            frame "SwitchToLog" {
              w396 = Mode_Enum."Logging" ("Operation.Operation Mode")
              n139 = call "File Dialog"("prompt"="Where do you want to log measurements?", "default name"="LogFile.csv", "pattern (all files)"="*.csv", "pattern label"="CSV file") -> ("selected path"=w385:path, "cancelled"=w389:bool)  [unwired: 8 in, 2 out]
              n140 = Bundle By Name(cluster=w398, "Operation.Operation Mode"=w396, "Operation.NewLog?"=TRUE) -> (w397:T7)
              n141 = case shown="\"Logging\", Default" w396 {
                tunnel: ["Measure and logging\n" "Off\n" "Measure only\n"] -> w395
                frame "Logging", Default {
                }
                frame "Idle-Off" {
                }
                frame "Idle" {
                }
              }
              n142 = control-ref of="Status"() -> (w390:refnum<vi>)
              n143 = Concatenate Strings("Changed Mode to: " ("string"), w395) -> (w393:string)
              n144 = property on="Logging" class="Bool (strict)"("Value"=TRUE ("Logging")) -> ()  [unwired: 2 in, 2 out]
              n145 = property on="Measuring" class="Bool (strict)"("Value"=TRUE ("Measuring")) -> ()  [unwired: 2 in, 2 out]
              n146 = call "GEN_WriteStatus.vi"("Input String"=w393, "error in (no error)"=w392, "Config_Cluster"=w397, "Status Ref"=w390) -> ("error out"=w391:errorcluster, "Config_Cluster Out"=w388:T7)  [unwired: 6 in]
              n147 = case shown="False" w389 {
                tunnel: w388 -> [w403 w405]
                tunnel: [w402 w405] -> w387
                tunnel: [GEN_States."RefreshMUnits" ("State") GEN_States."SwitchToMeas" ("State")] -> w386
                tunnel: w385 -> [w401 _]
                frame False {
                  n148 = Bundle By Name(cluster=w403, "General.Default Logging Path"=w401) -> (w402:T7)
                }
                frame True {
                }
              }
            }
            frame "UpdatePlots" {
              n149 = control-ref of="Test Graph"() -> (w418:refnum<vi>)
              n150 = call "LCR_PlotHelper.vi"("Y-Axis"="Y-Axis", "X-Axis"="X-Axis", "Data_IN"=w410, "Graph REF"=w418) -> ("Graph Out"=→"Test Graph":cluster{"Variant X":dbl, "Variant Y":dbl}[], "Data_Out"=w412:T5)  [unwired: 6 in]
              n151 = Unbundle By Name(w410) -> ("Scope Capture"=→"Scope Display":waveform(dbl))
            }
            frame "RefreshPlotMUnits" {
              n152 = control-ref of="Test Graph"() -> (w423:refnum<vi>)
              n153 = property on="Y-Axis" class="Enum (strict)"() -> ("Value"=w422:T2)  [unwired: 2 in, 2 out]
              n154 = property on="X-Axis" class="Enum (strict)"() -> ("Value"=w421:T2)  [unwired: 2 in, 2 out]
              n155 = call "LCR_PlotNamer.vi"("Y-Axis"=w422, "X-Axis"=w421, "Graph Ref In"=w423) -> ()  [unwired: 9 in]
            }
            frame "ClearBuffers" {
              n156 = in-place {
                n157 = in-place-cluster #1(w431) -> ("Measurements"=w436:T6[])
                n158 = Array Size(array=w436) -> (size(s)=w435:i32)
                n159 = Delete From Array(array=w436, length=w435, index=0) -> (array with subset deleted=w438:T6[])  [unwired: 1 out]
                n160 = in-place-cluster #1("Measurements"=w438) -> (w430:T5)
              }
            }
            frame "Disconnect" {
              n161 = Unbundle By Name(w454) -> ("Hardware.VISAS.SCOPE COM"=w440:refnum<visa-resource-name>, "Hardware.Global T VAR"=w457:refnum<k21>, "Hardware.Global B VAR"=w456:refnum<k21>)
              n162 = Enqueue Element At Opposite End(queue=w443, element=cluster{T3, bool} {enum."ApplyConfig", FALSE}) -> ()  [unwired: 2 in, 3 out]
              n163 = Close Variable Connection(11:w457) -> (0:w449:errorcluster)  [unwired: 1 in]
              n164 = VISA Close(VISA resource name=w440) -> (error out=w439:errorcluster)  [unwired: 1 in]
              n165 = Close Variable Connection(11:w456) -> (0:w450:errorcluster)  [unwired: 1 in]
              n166 = Merge Errors(w439, w449, w450) -> (w448:errorcluster)
              n167 = Unbundle By Name(w448) -> ("source"=w446:string)
              n168 = control-ref of="Status"() -> (w455:refnum<vi>)
              n169 = Concatenate Strings(w446, "\r", "Disconnected\n" ("string")) -> (w447:string)
              n170 = call "GEN_WriteStatus.vi"("Input String"=w447, "error in (no error)"=w452, "Config_Cluster"=w454, "Status Ref"=w455) -> ("error out"=w451:errorcluster, "Config_Cluster Out"=w453:T7)  [unwired: 6 in]
            }
            frame "ExitSafe" {
              n171 = Unbundle By Name(w472) -> ("Hardware.VISAS.SCOPE COM"=w461:refnum<visa-resource-name>, "Hardware.Global T VAR"=w475:refnum<k21>, "Hardware.Global B VAR"=w474:refnum<k21>)
              n172 = VISA Close(VISA resource name=w461) -> (error out=w460:errorcluster)  [unwired: 1 in]
              n173 = Close Variable Connection(11:w475) -> (0:w467:errorcluster)  [unwired: 1 in]
              n174 = Close Variable Connection(11:w474) -> (0:w468:errorcluster)  [unwired: 1 in]
              n175 = Merge Errors(w460, w467, w468) -> (w466:errorcluster)
              n176 = Unbundle By Name(w466) -> ("source"=w464:string)
              n177 = control-ref of="Status"() -> (w473:refnum<vi>)
              n178 = Concatenate Strings(w464, "\r", "Exit\n" ("string")) -> (w465:string)
              n179 = call "GEN_WriteStatus.vi"("Input String"=w465, "error in (no error)"=w470, "Config_Cluster"=w472, "Status Ref"=w473) -> ("error out"=w469:errorcluster, "Config_Cluster Out"=w471:T7)  [unwired: 6 in]
            }
          }
          n180 = Merge Errors(w94, w95) -> (w105:errorcluster)
          n181 = call "GEN_CulArray.vi"("Max Values"="Max Elements", "Data_Cluster"=w92) -> ("Data_Cluster Out"=w91:T5)  [unwired: 9 in]
          n182 = Or(x=w105, y=w104) -> (x .or. y?=w103:bool)
        }
      }
      frame Error {
      }
    }
  }
  n183 = property on="Measuring" class="Bool (strict)"("Colors [4]"=w3) -> ()  [unwired: 2 in, 2 out]
  n184 = property on="Logging" class="Bool (strict)"("Colors [4]"=w3) -> ()  [unwired: 2 in, 2 out]
  "Globals" <- FALSE ("Globals")
  "Scope" <- FALSE ("HM 8118")
  "Logging" <- FALSE ("Logging")
  "Measuring" <- FALSE ("Measuring")
  "Generator" <- FALSE ("Generator")
  "VNA" <- FALSE ("VNA")
